vi "Get Menu Items.vi"(8 "error in (no error)":errorcluster, 9 "GUID":string, 10 "Item Ref":T1 format="%.0x", 11 "System Explorer Dispatcher Implementation in":refnum<class "System Explorer Dispatcher Implementation.lvclass">) -> (0 "error out":errorcluster, 2 "Menu Items":string[](array[string]), 3 "System Explorer Dispatcher Implementation out":refnum<class "System Explorer Dispatcher Implementation.lvclass">)   [LabVIEW 2020, in "Communication Bus Template System Explorer.lvlib" / "Implementation.lvlib" / "System Explorer Dispatcher Implementation.lvclass"]
uses:
  System Explorer Dispatcher Implementation.lvclass
  <vilib>/NI VeriStand/Custom Device API/Custom Device Item Ref.ctl
  Scripting/Constants.vi
  Scripting/Communication Bus Template Scripting.lvlib
  <vilib>/NI VeriStand/Custom Device API/Custom Device API.lvlib
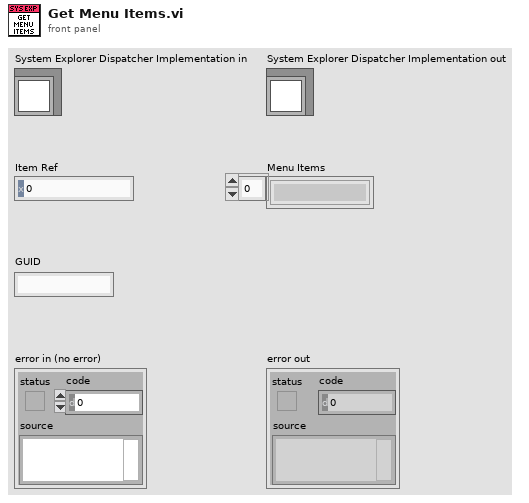
[diagram p1: front panel]
types:
  T1 = typedef "Custom Device API.lvlib/Custom Device Item Ref.ctl" = u64
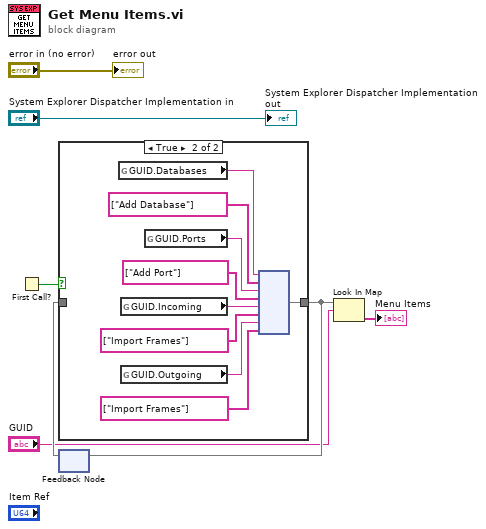
[diagram p0: block diagram]
diagram:
  n1 = First Call?() -> (First Call?: T/F=w5:bool)
  n2 = feedback #1() -> (w4:map{string, string[]})  [unwired: 1 in]
  n3 = case shown="True" w5 {
    tunnel: [w8 w17] -> w3
    tunnel: w4 -> [w8 _]
    frame False {
    }
    frame True {
      n4 = global read "Constants.vi" "GUID.Databases"() -> (w16:string)
      n5 = global read "Constants.vi" "GUID.Incoming"() -> (w12:string)
      n6 = global read "Constants.vi" "GUID.Outgoing"() -> (w10:string)
      n7 = global read "Constants.vi" "GUID.Ports"() -> (w15:string)
      n8 = node(w16, string[] ["Add Database"], w15, string[] ["Add Port"], w12, string[] ["Import Frames"], w10, string[] ["Import Frames"]) -> (w17:map{string, string[]})
    }
  }
  n9 = feedback-in #1(w3) -> ()
  n10 = Look In Map(map=w3, key="GUID") -> (value=→"Menu Items":string[])  [unwired: 1 in, 1 out]
  "error out" <- "error in (no error)"
  "System Explorer Dispatcher Implementation out" <- "System Explorer Dispatcher Implementation in"
